vi "Z6_Beamline.PC _Picture Condition Services.vi"(0 "i ref in":refnum<vi>, 2 "Instancename":string, 5 "error IO":errorcluster) -> (14 "i ref out":refnum<vi>, 19 "error out":errorcluster)   [LabVIEW 2014, in "Z6_Beamline.lvlib"]
doc: "This is a Proc Case of the Beamline Class."
uses:
  Z6_Beamline.lvlib
  PH_Common/Picture/PH_Picture.Alignment.ctl
  PH_Beamline_Common/PH_Beamline_Common.lvlib
  CSCore/CSSystem/CSSystemLib/CSSystemLib.lvlib
  PH_Common/PH_Common.lvlib
  PH_BL-Master/PH_BL-Master.lvlib
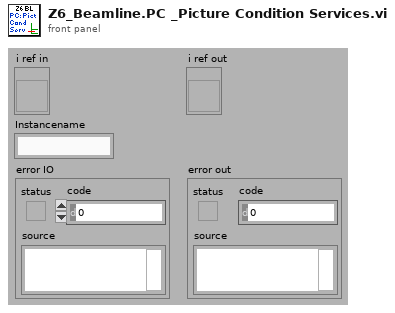
[diagram p1: front panel]
types:
  T1 = typedef "PH_BL-Master.lvlib/PH_BL-Master.i attribute.ctl" = cluster{"Remote controlled":bool, "Boolean Condition Service Subscriber":refnum<vi>[], "Picture Condition Service Subscriber":refnum<vi>[], "R2S":cluster{"GUI Ref":refnum<vi>, "State":bool}, "Vacua":cluster{"GUI Ref":refnum<vi>, "Limit":dbl, "Curr Value":dbl, "in range":bool}[], "O2 Inspection":cluster{"GUI Ref":refnum<vi>, "Concentration":dbl, "State":T2}[], "Boolean Status Service Subscriber":cluster{"GUI Ref":refnum<vi>, "Status":T2, "no Link?":bool, "Status Subscriber Class":T3}[], "Picture Status Service Subscriber":cluster{"GUI Ref":refnum<vi>, "Status":T2, "no Link?":bool, "Status Subscriber Class":T3}[], "6P 4Q Service Subscriber":cluster{"GUI Ref":refnum<vi>, "Selector":T4, "no Link?":bool}[], "Index of latest 6P 4Q changing Instance":i32, "Index of latest Picture Status changing Instance":i32, "Index of latest Boolean Status changing Instance":i32, "Vision ID on same Node":string, "Start Phase over?":bool, "GUI Ref Delete":refnum<vi>}
  T2 = typedef "PH_StatusHandler.lvlib/PH_StatusHandler.Status.ctl" = i16
  T3 = typedef "PH_BL-Master.lvlib/PH_BL-Master.Status Subscriber Class.ctl" = enum16{"unknown", "Switch", "BB", "6P Switch", "Switch GUI", "Switch and 6P State", "Force Sensor"}
  T4 = typedef "PH_4_Pos_Selector.lvlib/PH_4_Pos_Selector.Position Selector.ctl" = u16
  T5 = typedef "PH_Common.lvlib/PH_Picture.Alignment.ctl" = enum16{"neutral", "left", "right", "up", "down", "vertical", "horizontal", "left down to right up", "left up to right down"}
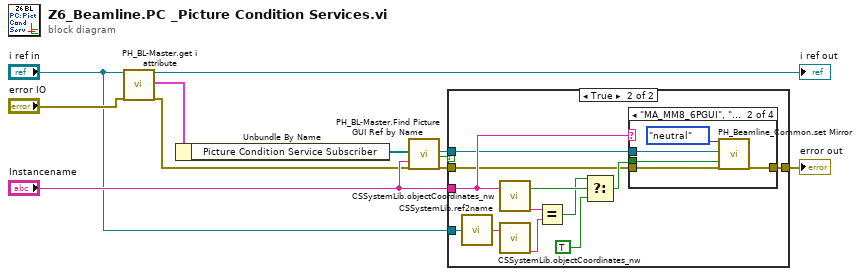
[diagram p0: block diagram]
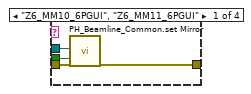
[diagram p3: hidden frame]
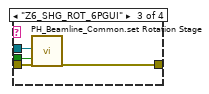
[diagram p4: hidden frame]
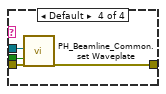
[diagram p5: hidden frame]
diagram:
  n1 = call "PH_BL-Master.get i attribute.vi"("i ref in"="i ref in", "error in (no error)"="error IO") -> ("i ref out"=→"i ref out":refnum<vi>, "i attribute"=w11:T1, "error out"=w3:errorcluster)  [unwired: 15 in]
  n2 = Unbundle By Name(w11) -> ("Picture Condition Service Subscriber"=w7:refnum<vi>[])
  n3 = call "PH_BL-Master.Find Picture GUI Ref by Name.vi"("Pic Ref Array"=w7, "Label"="Instancename", "error in"=w3) -> ("Wanted Pic GUI Ref"=w5:refnum<vi>, "Ref found?"=w4:bool, "error out"=w2:errorcluster)  [unwired: 13 in, 1 out]
  n4 = case shown="True" w4 {
    tunnel: [w12 w24] -> w9
    tunnel: "Instancename" -> [_ w15]
    tunnel: "i ref in" -> [_ w16]
    tunnel: w5 -> [_ w14]
    tunnel: w2 -> [w12 w13]
    frame False {
    }
    frame True {
      n5 = call "CSSystemLib.ref2name.vi"("obj refnum"=w16) -> ("name"=w18:string)
      n6 = call "CSSystemLib.objectCoordinates_nw.vi"("name"=w15) -> ("obj exists"=w23:bool, "node"=w22:string)  [unwired: 15 in, 2 out]
      n7 = call "CSSystemLib.objectCoordinates_nw.vi"("name"=w18) -> ("node"=w21:string)  [unwired: 15 in, 3 out]
      n8 = Equal?(x=w22, y=w21) -> (x = y?=w20:bool)
      n9 = Select(t=w20, s=w23, f=TRUE) -> (s? t:f=w17:bool)
      n10 = case shown="\"MA_MM8_6PGUI\", \"MA_MM9_6PGUI\", \"Z6_SHG_TIP-TILT_6PGUI\"" w15 {
        tunnel: w14 -> [w27 w32 w36 w41]
        tunnel: [w28 w33 w37 w40] -> w24
        tunnel: w17 -> [w26 w31 w35 w39]
        tunnel: w13 -> [w25 w29 w34 w38]
        frame "Z6_MM10_6PGUI", "Z6_MM11_6PGUI" {
          n11 = call "PH_Beamline_Common.set Mirror.vi"("CtlRef"=w27, "GUI Instance does not exist or here?"=w26, "error in (no error)"=w25) -> ("error out"=w28:errorcluster)  [unwired: 16 in]
        }
        frame "MA_MM8_6PGUI", "MA_MM9_6PGUI", "Z6_SHG_TIP-TILT_6PGUI" {
          n12 = call "PH_Beamline_Common.set Mirror.vi"("Alignment (left down to right up)"=PH_Picture.Alignment."neutral", "CtlRef"=w32, "GUI Instance does not exist or here?"=w31, "error in (no error)"=w29) -> ("error out"=w33:errorcluster)  [unwired: 15 in]
        }
        frame "Z6_SHG_ROT_6PGUI" {
          n13 = call "PH_Beamline_Common.set Rotation Stage.vi"("CtlRef"=w36, "GUI Instance does not exist or here?"=w35, "error in (no error)"=w34) -> ("error out"=w37:errorcluster)  [unwired: 16 in]
        }
        frame Default {
          n14 = call "PH_Beamline_Common.set Waveplate.vi"("CtlRef"=w41, "GUI Instance does not exist or here?"=w39, "error in (no error)"=w38) -> ("error out"=w40:errorcluster)  [unwired: 16 in]
        }
      }
    }
  }
  "error out" <- w9
